vi "Sample_Prod-Cons.vi"() -> ()   [LabVIEW 2022 SP3]
uses:
  4652784b-b2c9-4b62-9975-14206a9570d8.vi
panel:
  in  "Gen. Test Error":bool
  in  "Interloop Stop":bool
  out "State":string
  in  "Stop":bool
  in  "Action":bool
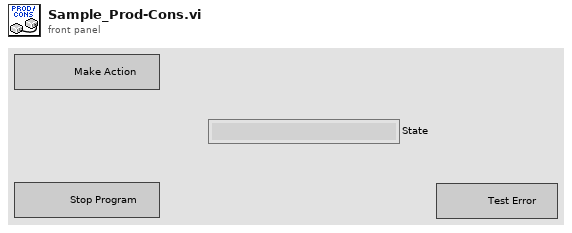
[diagram p1: front panel]
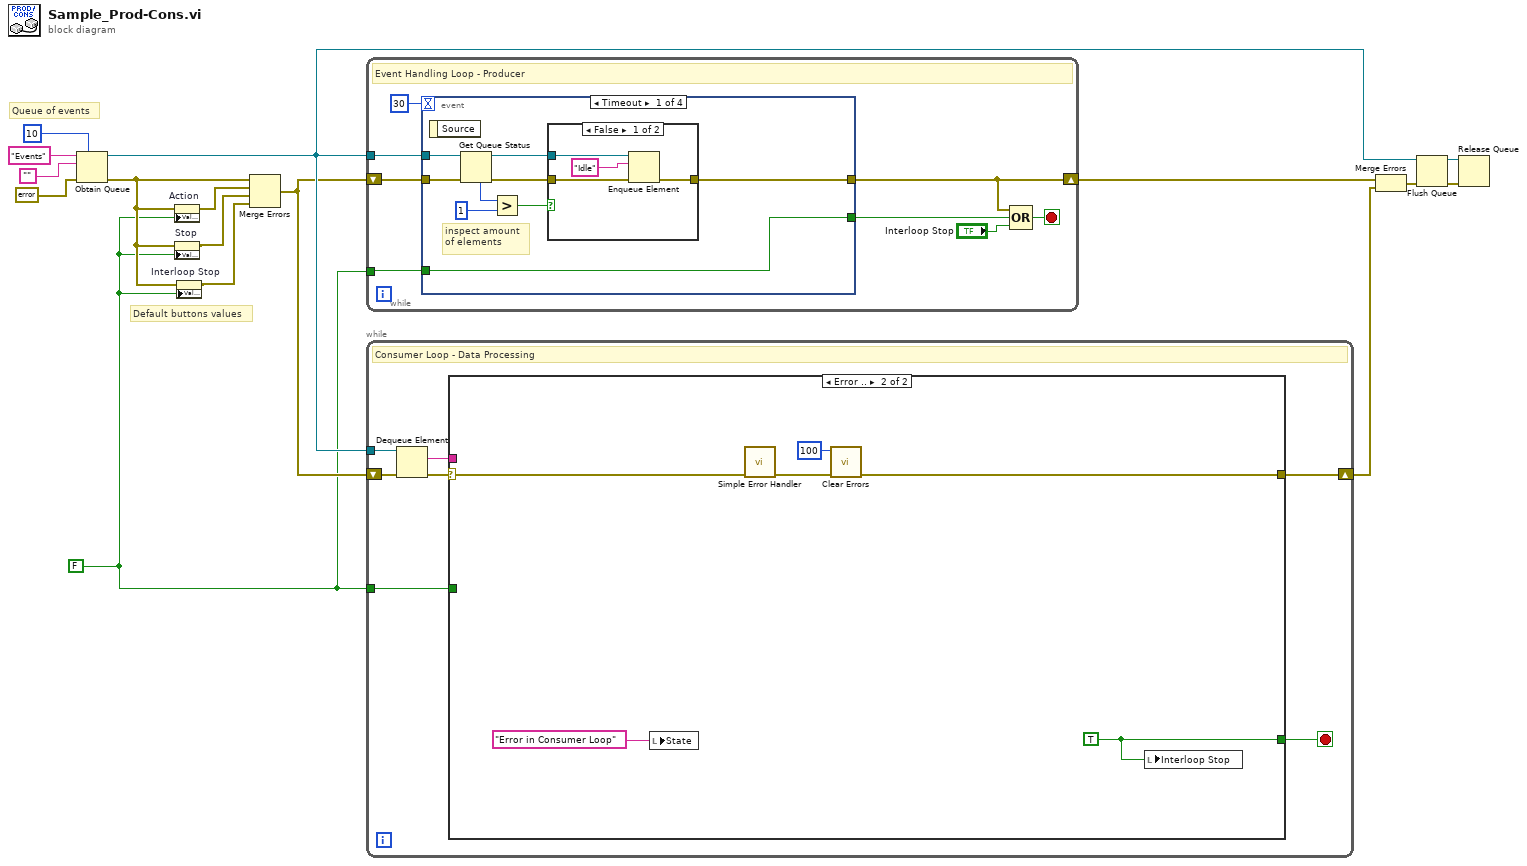
[diagram p0: block diagram]
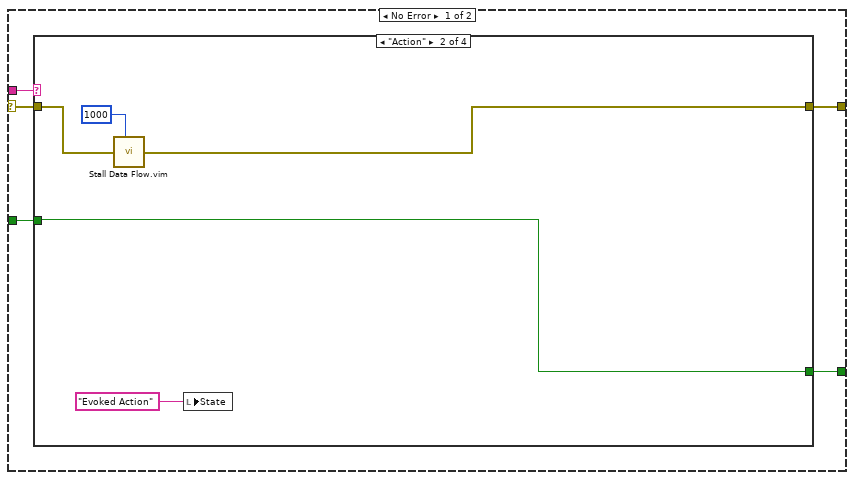
[diagram p2: hidden frame]
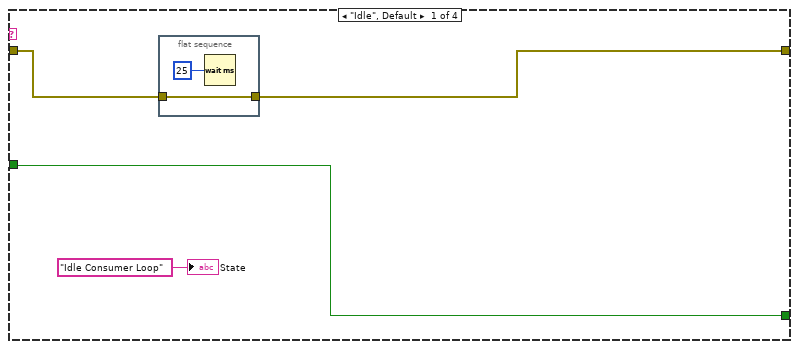
[diagram p3: hidden frame]
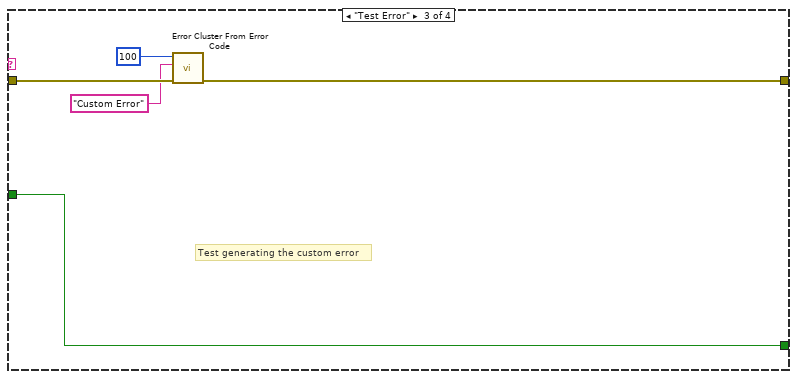
[diagram p4: hidden frame]
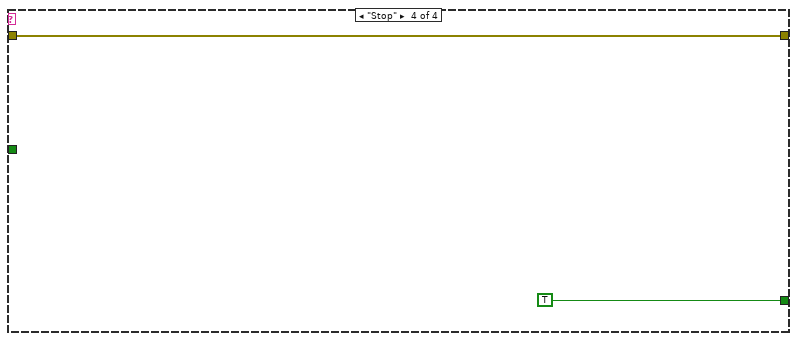
[diagram p5: hidden frame]
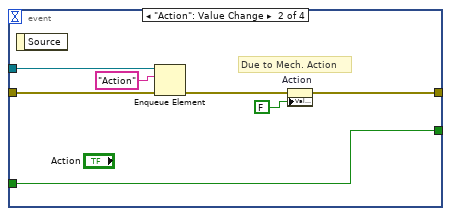
[diagram p7: hidden frame]
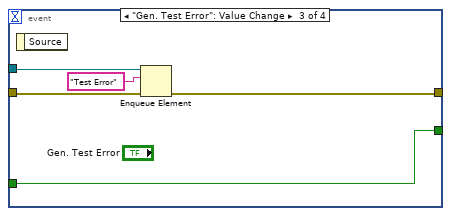
[diagram p8: hidden frame]
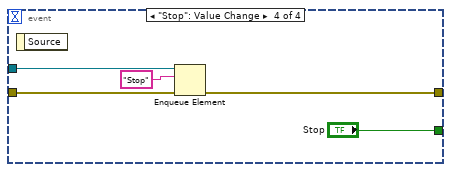
[diagram p9: hidden frame]
diagram:
  w2 = FALSE
  # "Default buttons values"
  # "Queue of events"
  n1 = Obtain Queue(max queue size (-1, unlimited)=10, name (unnamed)="Events", element data type="", error in (no error)=errorcluster {"status"=FALSE, "code"=0, "source"=""}) -> (queue out=w10:refnum<queue>, error out=w3:errorcluster)  [unwired: 1 in, 1 out]
  n2 = property on="Action" class="Bool (strict)"(error in=w3, "Value"=w2) -> (error out=w6:errorcluster)  [unwired: 1 in, 1 out]
  n3 = property on="Stop" class="Bool (strict)"(error in=w3, "Value"=w2) -> (error out=w4:errorcluster)  [unwired: 1 in, 1 out]
  n4 = property on="Interloop Stop" class="Bool (strict)"(error in=w3, "Value"=w2) -> (error out=w1:errorcluster)  [unwired: 1 in, 1 out]
  n5 = Merge Errors(w3, w6, w4, w1) -> (w5:errorcluster)
  n6 = while {
    tunnel: w10 -> [w23]
    shift-right: [w19] -> w14
    shift-left: w5 -> [w22]
    tunnel: w2 -> [w21]
    stop <- w18 stop-if-true
    # "Event Handling Loop - Producer"
    n7 = event shown="[0] Timeout" {
      selector: _ -> [_ _ _ _]
      dyn-events: _ -> [_ _ _ _]
      timeout: 30 -> [_ _ _ _]
      tunnel: w23 -> [w33 w44 w48 w53]
      tunnel: w22 -> [w32 w45 w47 w54]
      tunnel: [w26 w40 w46 w51] -> w19
      tunnel: [w25 w42 w50 "Stop"] -> w20
      tunnel: w21 -> [w25 w42 w50 _]
      event Timeout {
        # "inspect amount\nof elements"
        n8 = event-data() -> ()  [unwired: 1 in, 1 out]
        n9 = Get Queue Status(queue=w33, error in (no error)=w32) -> (queue out=w29:refnum<queue>, error out=w28:errorcluster, # elements in queue=w31:i32)  [unwired: 1 in, 5 out]
        n10 = Greater?(x=w31, y=1) -> (0:w27:bool)
        n11 = case shown="False" w27 {
          tunnel: w29 -> [w37 _]
          tunnel: w28 -> [w35 w38]
          tunnel: [w34 w38] -> w26
          frame False {
            n12 = Enqueue Element(queue=w37, element="Idle", error in (no error)=w35) -> (error out=w34:errorcluster)  [unwired: 1 in, 2 out]
          }
          frame True {
          }
        }
      }
      event "Action": Value Change {
        # "Due to Mech. Action"
        n13 = event-data() -> ()  [unwired: 1 in, 1 out]
        n14 = Enqueue Element(queue=w44, element="Action", error in (no error)=w45) -> (error out=w41:errorcluster)  [unwired: 1 in, 2 out]
        n15 = property on="Action" class="Bool (strict)"(error in=w41, "Value"=FALSE ("Action")) -> (error out=w40:errorcluster)  [unwired: 1 in, 1 out]
      }
      event "Gen. Test Error": Value Change {
        n16 = event-data() -> ()  [unwired: 1 in, 1 out]
        n17 = Enqueue Element(queue=w48, element="Test Error", error in (no error)=w47) -> (error out=w46:errorcluster)  [unwired: 1 in, 2 out]
      }
      event "Stop": Value Change {
        n18 = event-data() -> ()  [unwired: 1 in, 1 out]
        n19 = Enqueue Element(queue=w53, element="Stop", error in (no error)=w54) -> (error out=w51:errorcluster)  [unwired: 1 in, 2 out]
      }
    }
    n20 = Compound Arithmetic op=OR(w19, w20, "Interloop Stop") -> (w18:bool)
  }
  n21 = while {
    tunnel: w10 -> [w62]
    tunnel: w2 -> [w57]
    shift-right: [w58] -> w13
    shift-left: w5 -> [w61]
    stop <- w59 stop-if-true
    # "Consumer Loop - Data Processing"
    n22 = Dequeue Element(queue=w62, error in (no error)=w61) -> (element=w60:string, error out=w56:errorcluster)  [unwired: 1 in, 2 out]
    n23 = case shown="Error .." w56 {
      selector: w56 -> [w63 w89]
      tunnel: w60 -> [w67 _]
      tunnel: [w66 w91] -> w59
      tunnel: [w65 w86] -> w58
      tunnel: w57 -> [w64 _]
      frame No Error {
        n24 = case shown="\"Action\"" w67 {
          tunnel: w63 -> [w69 w77 w82 w84]
          tunnel: [w68 w74 w83 TRUE] -> w66
          tunnel: [w70 w75 w79 w84] -> w65
          tunnel: w64 -> [w68 w74 w83 _]
          frame "Idle", Default {
            n25 = flat-sequence {
              tunnel: w69 -> [w72]
              tunnel: [w72] -> w70
              frame #0 {
                n26 = Wait (ms)(milliseconds to wait=u32 25) -> ()  [unwired: 1 out]
              }
            }
            "State" <- "Idle Consumer Loop" ("Answer")
          }
          frame "Action" {
            n27 = call "Stall Data Flow.vim"("value in"=w77, "milliseconds to wait"=u32 1000) -> ("value out"=w75:errorcluster)  [unwired: 1 out]
            n28 = local write "State"("Evoked Action" ("Answer")) -> ()
          }
          frame "Test Error" {
            # "Test generating the custom error"
            n29 = call <vilib>:"Error Cluster From Error Code.vi"("error in (no error)"=w82, "error message (\"\")"="Custom Error" ("error message (\"\")"), "error code (0)"=100) -> ("error out"=w79:errorcluster)  [unwired: 6 in]
          }
          frame "Stop" {
          }
        }
      }
      frame Error {
        w91 = TRUE
        n30 = local write "State"("Error in Consumer Loop" ("State")) -> ()
        n31 = call <vilib>:"Simple Error Handler.vi"("error in (no error)"=w89) -> ("error out"=w87:errorcluster)  [unwired: 4 in, 4 out]
        n32 = call <vilib>:"Clear Errors.vi"("error in (no error)"=w87, "specific error code to clear (0: all)"=100) -> ("error out"=w86:errorcluster)  [unwired: 4 in, 1 out]
        n33 = local write "Interloop Stop"(w91) -> ()
      }
    }
  }
  n34 = Merge Errors(w14, w13) -> (w11:errorcluster)
  n35 = Flush Queue(queue=w10, error in (no error)=w11) -> (queue out=w8:refnum<queue>, error out=w9:errorcluster)  [unwired: 1 out]
  n36 = Release Queue(queue=w8, error in (no error)=w9) -> ()  [unwired: 1 in, 3 out]
